vi "Run Filter.vi"(8 "error in (no error)":errorcluster, 10 "resource entries in":T1(array[cluster]) {"FPGA CD Ref" format="%.0x"; "reserver" format="%.0x"}, 11 "Input Type Filter in":refnum<class "Input Type Filter.lvclass">) -> (0 "error out":errorcluster, 2 "resource entries out":T1(array[cluster]) {"FPGA CD Ref" format="%.0x"; "reserver" format="%.0x"})   [LabVIEW 2016, in "FPGA Resource Manager.lvlib" / "Input Type Filter.lvclass"]
uses:
  FPGA RM Test Client Configuration.llb/Input Type Filter.lvclass
  FPGA RM Test Client Configuration.llb/Input Type Filter.lvclass/Input Type Filter.ctl
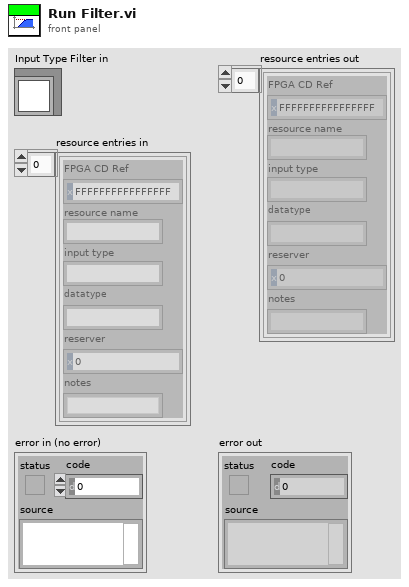
[diagram p1: front panel]
types:
  T1 = cluster{"FPGA CD Ref":u64, "resource name":string, "input type":string, "datatype":string, "reserver":u64, "notes":string}[]
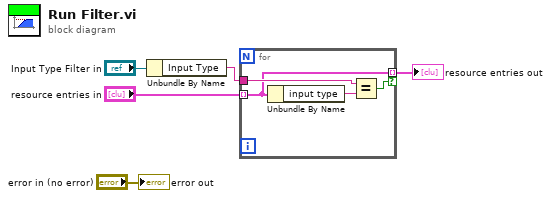
[diagram p0: block diagram]
diagram:
  n1 = Unbundle By Name("Input Type Filter in") -> ("Input Type"=w4:string)
  n2 = for {
    tunnel: w4 -> [w9]
    tunnel: "resource entries in" -> [w7] mode=indexing
    tunnel: [w7] -> w2 mode=indexing if=w6
    n3 = Unbundle By Name(w7) -> ("input type"=w8:string)
    n4 = Equal?(x=w9, y=w8) -> (x = y?=w6:bool)
  }
  "resource entries out" <- w2
  "error out" <- "error in (no error)"
